vi "Open Config File.vi"(8 "error in (no error)":errorcluster, 10 "Config File Path":path, 11 "Database in":refnum<class "Database.lvclass">) -> (0 "error out":errorcluster, 3 "Database out":refnum<class "Database.lvclass">)   [LabVIEW 2015, in "Database.lvlib" / "Database.lvclass"]
uses:
  Database.lvclass
  Database.lvclass/Database.ctl
  <vilib>/Utility/config.llb/NI_LVConfig.lvlib
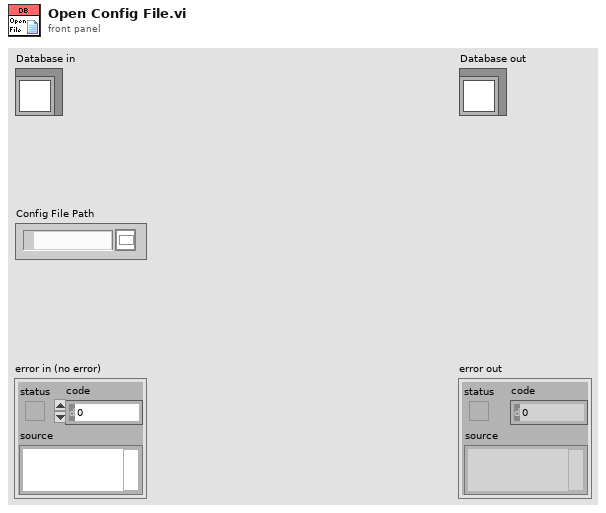
[diagram p1: front panel]
types:
  T1 = typedef "NI_LVConfig.lvlib/Config Data RefNum.ctl" = refnum<k1>
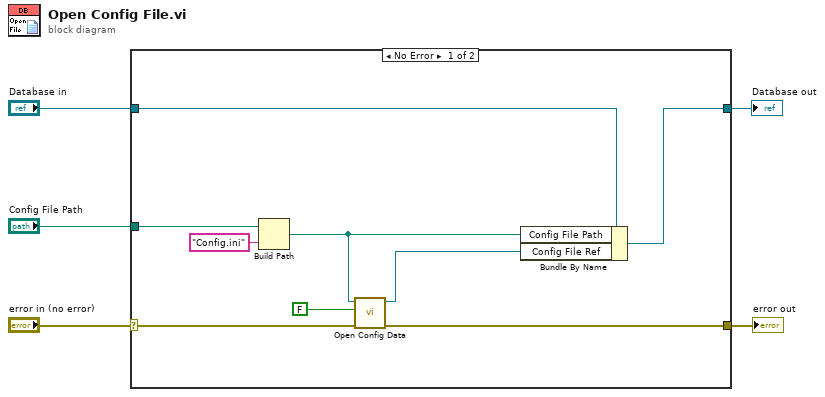
[diagram p0: block diagram]
diagram:
  n1 = case shown="No Error" "error in (no error)" {
    selector: "error in (no error)" -> [w13 w16]
    tunnel: [w12 w16] -> w4
    tunnel: [w9 w15] -> w2
    tunnel: "Database in" -> [w14 w15]
    tunnel: "Config File Path" -> [w10 _]
    frame No Error {
      n2 = Build Path(base path=w10, name or relative path="Config.ini") -> (appended path=w8:path)
      n3 = call <vilib>:"Open Config Data.vi"("error in (no error)"=w13, "create file if necessary (T)"=FALSE, "configuration file path"=w8) -> ("error out"=w12:errorcluster, "refnum"=w7:T1)  [unwired: 6 in, 1 out]
      n4 = Bundle By Name(cluster=w14, "Config File Path"=w8, "Config File Ref"=w7) -> (w9:refnum<class "Database.lvclass">)
    }
    frame Error {
    }
  }
  "error out" <- w4
  "Database out" <- w2
